vi "Get Available Sections.vi"(8 "error in (no error)":errorcluster, 11 "Session in":refnum<k21>) -> (0 "error out":errorcluster, 2 "Sections":T1[](array[typedef]) {"Visibility Type" items=["standard", "hidden", "system", "unknown", "startup", "image"]}, 3 "Session out":refnum<k21>)   [LabVIEW 2014, in "nisyscfg.lvlib"]
uses:
  nisyscfg.lvlib
  Software Extended.ctl
  Component Type.ctl
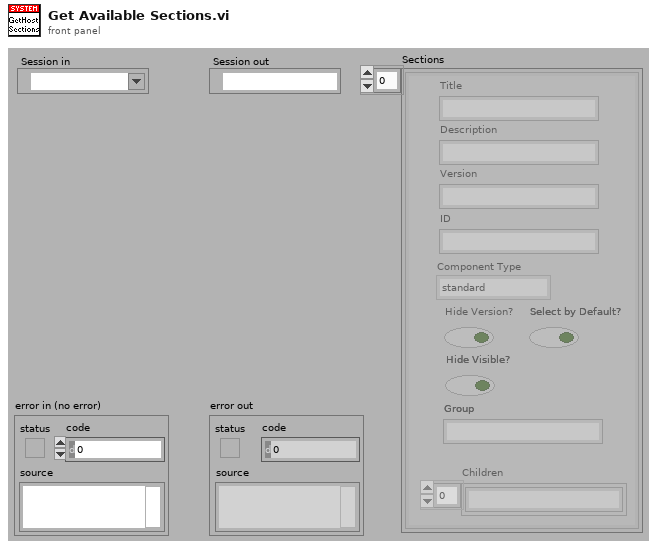
[diagram p1: front panel]
types:
  T1 = typedef "nisyscfg.lvlib/Software Extended.ctl" = cluster{"Description":string, "ID":string, "Version":string, "Title":string, "Visibility Type":T2, "Hide Version?":bool, "Children":string[], "Select by Default?":bool, "Hide Visible?":bool, "Group":string}
  T2 = typedef "nisyscfg.lvlib/Component Type.ctl" = u32
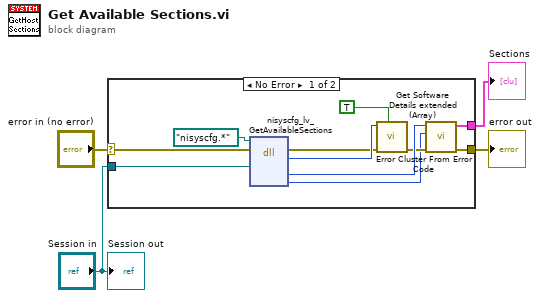
[diagram p0: block diagram]
diagram:
  n1 = case shown="No Error" "error in (no error)" {
    selector: "error in (no error)" -> [w13 w16]
    tunnel: [w7 w16] -> w4
    tunnel: "Session in" -> [w12 _]
    tunnel: [w6 _] -> w1
    frame No Error {
      n2 = dll-call lib="nisyscfg.*" fn="nisyscfg_lv_GetAvailableSections" label="GetAvailableSections"(path in=path "nisyscfg.*", error in=w13, "system"=w12) -> (error out=w14:errorcluster, "result"=w15:i32, "sections"=w9:u64, "numSections"=w5:i32)  [unwired: 4 in, 1 out]
      n3 = call "Error Cluster From Error Code.vi"("show call chain? (False)"=TRUE, "error in (no error)"=w14, "error code (0)"=w15) -> ("error out"=w8:errorcluster)  [unwired: 6 in]
      n4 = call "Get Software Details extended (Array).vi"("error in (no error)"=w8, "Number of Elements"=w5, "Enumerator in"=w9) -> ("error out"=w7:errorcluster, "Software Components"=w6:T1[])  [unwired: 7 in]
    }
    frame Error {
    }
  }
  "error out" <- w4
  "Sections" <- w1
  "Session out" <- "Session in"
